vi "Untitled 1.vi"   [LabVIEW 2024]
uses:
  Libraries/Inversor/Inversor.lvlib
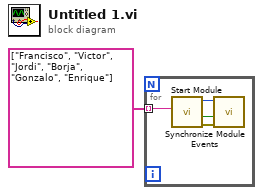
[diagram p0: block diagram]
diagram:
  n1 = for {
    tunnel: string[] ["Francisco", "Victor", "Jordi", "Borja", "Gonzalo", "Enrique"] ("Nombre") -> [w2] mode=indexing
    n2 = call "Start Module.vi"("Nombre"=w2) -> ("error out"=w4:errorcluster, "Wait for Event Sync?"=w5:bool, "Module ID"=w3:i32)  [unwired: 6 in, 2 out]
    n3 = call "Synchronize Module Events.vi"("error in"=w4, "Wait for Event Sync?"=w5, "Module ID in"=w3) -> ()  [unwired: 7 in, 2 out]
  }
